vi "Flatten Value.vi"(8 "error in (no error)":errorcluster, 11 "Boolean in":refnum<class "Path Builder.lvclass">) -> (0 "error out":errorcluster, 2 "Value":string, 3 "Boolean out":refnum<class "Path Builder.lvclass">)   [LabVIEW 2017, in "Custom Type Test Executive.lvlib" / "Path Builder.lvclass"]
uses:
  <vilib>/gpm_packages/@cs/test-executive/Source/Custom Type Test Executive/Path Builder Data Type/Path Builder.lvclass
  <vilib>/gpm_packages/@cs/test-executive/Source/Custom Type Test Executive/Path Builder Data Type/Path Builder.lvclass/Path Builder.ctl
  <vilib>/gpm_packages/@cs/test-executive/Source/Path Builder/IPath Builder/IPath Builder.lvclass
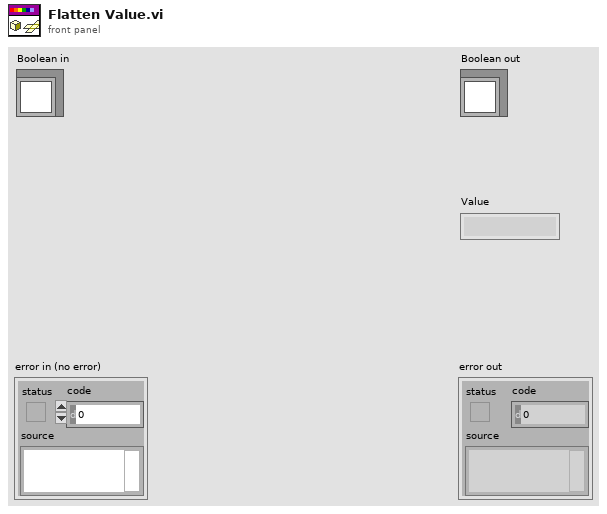
[diagram p1: front panel]
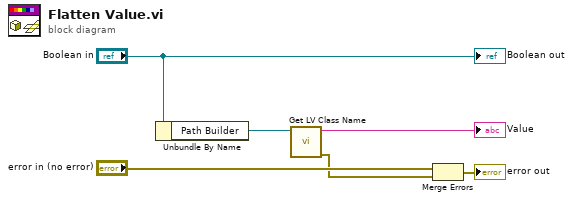
[diagram p0: block diagram]
diagram:
  n1 = Unbundle By Name("Boolean in") -> ("Path Builder"=w3:refnum<class "IPath Builder.lvclass">)
  n2 = call <vilib>:"Get LV Class Name.vi"("object"=w3) -> ("error out"=w1:errorcluster, "class name"=→"Value":string)  [unwired: 9 in]
  n3 = Merge Errors("error in (no error)", w1) -> (→"error out":errorcluster)
  "Boolean out" <- "Boolean in"
